vi "CRYAutoScale Change.vi"(9 "sOption":string, 10 "Graph VI Ref":refnum<vi>, 11 "sAction":string) -> ()   [LabVIEW 2013]
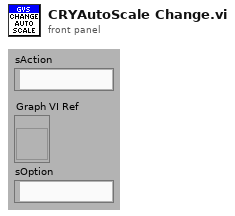
[diagram p1: front panel]
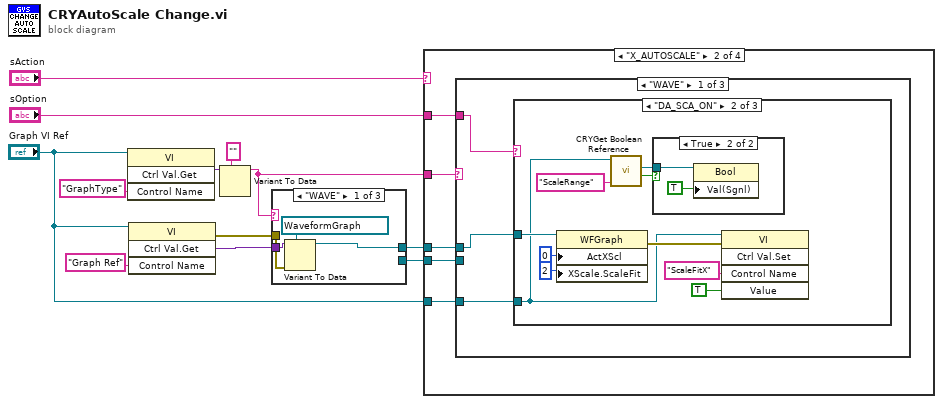
[diagram p0: block diagram]
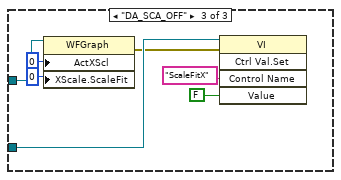
[diagram p5: hidden frame]
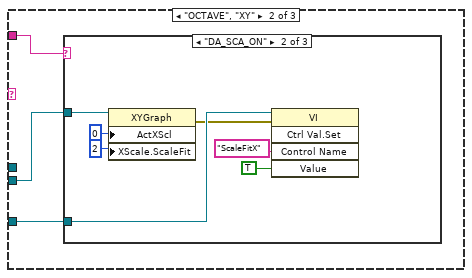
[diagram p6: hidden frame]
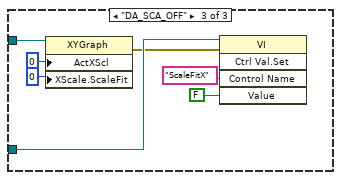
[diagram p8: hidden frame]
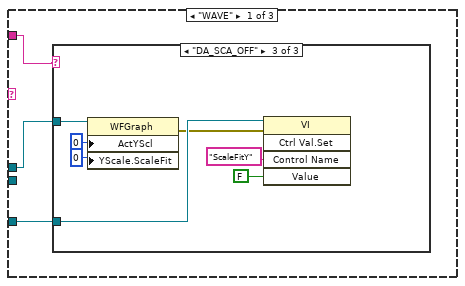
[diagram p11: hidden frame]
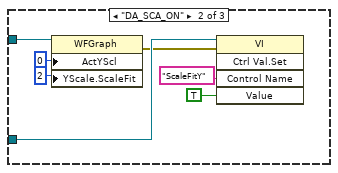
[diagram p13: hidden frame]
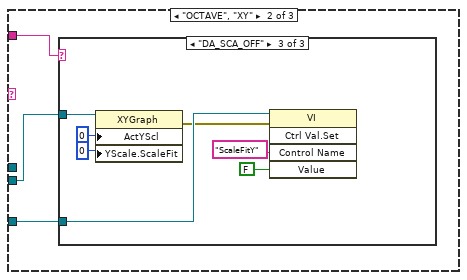
[diagram p14: hidden frame]
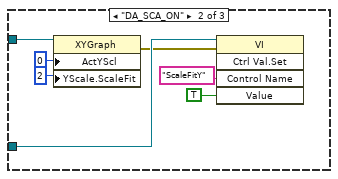
[diagram p16: hidden frame]
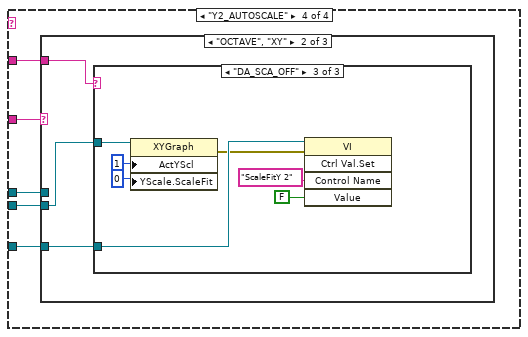
[diagram p17: hidden frame]
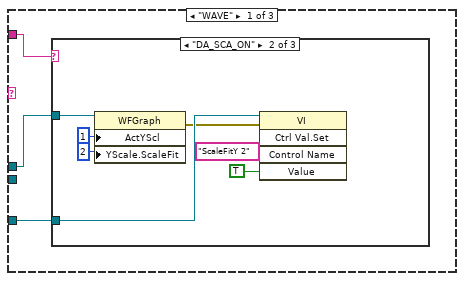
[diagram p18: hidden frame]
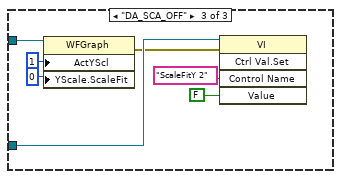
[diagram p20: hidden frame]
diagram:
  n1 = invoke class="VI" method="Ctrl Val.Get"(reference="Graph VI Ref", "Control Name"="GraphType") -> ("Get Control Value Variant"=w8:variant)  [unwired: 2 in, 3 out]
  n2 = invoke class="VI" method="Ctrl Val.Get"(reference="Graph VI Ref", "Control Name"="Graph Ref") -> (error out=w11:errorcluster, "Get Control Value Variant"=w12:variant)  [unwired: 2 in, 2 out]
  n3 = Variant To Data(type="" ("Control Name"), Variant=w8) -> (data=w4:string)  [unwired: 1 in, 1 out]
  n4 = case shown="\"WAVE\"" w4 {
    tunnel: w12 -> [w16 w20 _]
    tunnel: w11 -> [w15 w19 _]
    tunnel: [w13 _ _] -> w5
    tunnel: [_ w17 _] -> w3
    frame "WAVE" {
      n5 = Variant To Data(error in=w15, type=refnum<vi> refnum ("Legend Ref"), Variant=w16) -> (data=w13:refnum<vi>)  [unwired: 1 out]
    }
    frame "OCTAVE", "XY" {
      n6 = Variant To Data(error in=w19, type=refnum<vi> refnum ("Legend Ref"), Variant=w20) -> (data=w17:refnum<vi>)  [unwired: 1 out]
    }
    frame Default {
    }
  }
  n7 = case shown="\"X_AUTOSCALE\"" "sAction" {
    tunnel: w5 -> [_ w24 w68 w107]
    tunnel: w4 -> [_ w25 w69 w108]
    tunnel: w3 -> [_ w23 w67 w106]
    tunnel: "sOption" -> [_ w22 w66 w105]
    tunnel: "Graph VI Ref" -> [_ w21 w65 w104]
    frame Default {
    }
    frame "X_AUTOSCALE" {
      n8 = case shown="\"WAVE\"" w25 {
        tunnel: w24 -> [w27 _ _]
        tunnel: w23 -> [_ w50 _]
        tunnel: w22 -> [w28 w49 _]
        tunnel: w21 -> [w26 w48 _]
        frame "WAVE" {
          n9 = case shown="\"DA_SCA_ON\"" w28 {
            tunnel: w27 -> [_ w37 w45]
            tunnel: w26 -> [_ w32 w42]
            frame "NONE", Default {
            }
            frame "DA_SCA_ON" {
              n10 = property class="WFGraph"(reference=w37, "ActXScl"=0 ("Active X Scale"), "XScale.ScaleFit"=u8 2 ("t")) -> (error out=w33:errorcluster)  [unwired: 1 in, 1 out]
              n11 = call "CRYGet Boolean Reference.vi"("Label Name"="ScaleRange" ("Control Name"), "VI Refnum"=w32) -> ("Exist?"=w30:bool, "Boolean Ref"=w29:refnum<vi>)  [unwired: 7 in, 1 out]
              n12 = case shown="True" w30 {
                tunnel: w29 -> [_ w40]
                frame False {
                }
                frame True {
                  n13 = property class="Bool"(reference=w40, "Val(Sgnl)"=TRUE ("Visible")) -> ()  [unwired: 1 in, 2 out]
                }
              }
              n14 = invoke class="VI" method="Ctrl Val.Set"(reference=w32, error in=w33, "Control Name"="ScaleFitX", "Value"=TRUE ("Visible")) -> ()  [unwired: 1 in, 5 out]
            }
            frame "DA_SCA_OFF" {
              n15 = property class="WFGraph"(reference=w45, "ActXScl"=0 ("Active X Scale"), "XScale.ScaleFit"=u8 0 ("t")) -> (error out=w41:errorcluster)  [unwired: 1 in, 1 out]
              n16 = invoke class="VI" method="Ctrl Val.Set"(reference=w42, error in=w41, "Control Name"="ScaleFitX", "Value"=FALSE ("Visible")) -> ()  [unwired: 1 in, 5 out]
            }
          }
        }
        frame "OCTAVE", "XY" {
          n17 = case shown="\"DA_SCA_ON\"" w49 {
            tunnel: w50 -> [_ w56 w62]
            tunnel: w48 -> [_ w52 w59]
            frame "NONE", Default {
            }
            frame "DA_SCA_ON" {
              n18 = property class="XYGraph"(reference=w56, "ActXScl"=0 ("Active X Scale"), "XScale.ScaleFit"=u8 2 ("t")) -> (error out=w51:errorcluster)  [unwired: 1 in, 1 out]
              n19 = invoke class="VI" method="Ctrl Val.Set"(reference=w52, error in=w51, "Control Name"="ScaleFitX", "Value"=TRUE ("Visible")) -> ()  [unwired: 1 in, 5 out]
            }
            frame "DA_SCA_OFF" {
              n20 = property class="XYGraph"(reference=w62, "ActXScl"=0 ("Active X Scale"), "XScale.ScaleFit"=u8 0 ("t")) -> (error out=w58:errorcluster)  [unwired: 1 in, 1 out]
              n21 = invoke class="VI" method="Ctrl Val.Set"(reference=w59, error in=w58, "Control Name"="ScaleFitX", "Value"=FALSE ("Visible")) -> ()  [unwired: 1 in, 5 out]
            }
          }
        }
        frame Default {
        }
      }
    }
    frame "Y1_AUTOSCALE" {
      n22 = case shown="Default" w69 {
        tunnel: w68 -> [w71 _ _]
        tunnel: w67 -> [_ w87 _]
        tunnel: w66 -> [w72 w88 _]
        tunnel: w65 -> [w70 w89 _]
        frame "WAVE" {
          n23 = case shown="\"DA_SCA_OFF\"" w72 {
            tunnel: w71 -> [_ w78 w84]
            tunnel: w70 -> [_ w74 w81]
            frame "NONE", Default {
            }
            frame "DA_SCA_ON" {
              n24 = property class="WFGraph"(reference=w78, "ActYScl"=0 ("Active X Scale"), "YScale.ScaleFit"=u8 2 ("t")) -> (error out=w73:errorcluster)  [unwired: 1 in, 1 out]
              n25 = invoke class="VI" method="Ctrl Val.Set"(reference=w74, error in=w73, "Control Name"="ScaleFitY", "Value"=TRUE ("Visible")) -> ()  [unwired: 1 in, 5 out]
            }
            frame "DA_SCA_OFF" {
              n26 = property class="WFGraph"(reference=w84, "ActYScl"=0 ("Active X Scale"), "YScale.ScaleFit"=u8 0 ("t")) -> (error out=w80:errorcluster)  [unwired: 1 in, 1 out]
              n27 = invoke class="VI" method="Ctrl Val.Set"(reference=w81, error in=w80, "Control Name"="ScaleFitY", "Value"=FALSE ("Visible")) -> ()  [unwired: 1 in, 5 out]
            }
          }
        }
        frame "OCTAVE", "XY" {
          n28 = case shown="\"DA_SCA_OFF\"" w88 {
            tunnel: w87 -> [_ w95 w101]
            tunnel: w89 -> [_ w91 w98]
            frame "NONE", Default {
            }
            frame "DA_SCA_ON" {
              n29 = property class="XYGraph"(reference=w95, "ActYScl"=0 ("Active X Scale"), "YScale.ScaleFit"=u8 2 ("t")) -> (error out=w90:errorcluster)  [unwired: 1 in, 1 out]
              n30 = invoke class="VI" method="Ctrl Val.Set"(reference=w91, error in=w90, "Control Name"="ScaleFitY", "Value"=TRUE ("Visible")) -> ()  [unwired: 1 in, 5 out]
            }
            frame "DA_SCA_OFF" {
              n31 = property class="XYGraph"(reference=w101, "ActYScl"=0 ("Active X Scale"), "YScale.ScaleFit"=u8 0 ("t")) -> (error out=w97:errorcluster)  [unwired: 1 in, 1 out]
              n32 = invoke class="VI" method="Ctrl Val.Set"(reference=w98, error in=w97, "Control Name"="ScaleFitY", "Value"=FALSE ("Visible")) -> ()  [unwired: 1 in, 5 out]
            }
          }
        }
        frame Default {
        }
      }
    }
    frame "Y2_AUTOSCALE" {
      n33 = case shown="\"OCTAVE\", \"XY\"" w108 {
        tunnel: w107 -> [w110 _ _]
        tunnel: w106 -> [_ w127 _]
        tunnel: w105 -> [w111 w128 _]
        tunnel: w104 -> [w109 w126 _]
        frame "WAVE" {
          n34 = case shown="\"DA_SCA_ON\"" w111 {
            tunnel: w110 -> [_ w117 w123]
            tunnel: w109 -> [_ w113 w120]
            frame "NONE", Default {
            }
            frame "DA_SCA_ON" {
              n35 = property class="WFGraph"(reference=w117, "ActYScl"=1 ("Active X Scale"), "YScale.ScaleFit"=u8 2 ("t")) -> (error out=w112:errorcluster)  [unwired: 1 in, 1 out]
              n36 = invoke class="VI" method="Ctrl Val.Set"(reference=w113, error in=w112, "Control Name"="ScaleFitY 2", "Value"=TRUE ("Visible")) -> ()  [unwired: 1 in, 5 out]
            }
            frame "DA_SCA_OFF" {
              n37 = property class="WFGraph"(reference=w123, "ActYScl"=1 ("Active X Scale"), "YScale.ScaleFit"=u8 0 ("t")) -> (error out=w119:errorcluster)  [unwired: 1 in, 1 out]
              n38 = invoke class="VI" method="Ctrl Val.Set"(reference=w120, error in=w119, "Control Name"="ScaleFitY 2", "Value"=FALSE ("Visible")) -> ()  [unwired: 1 in, 5 out]
            }
          }
        }
        frame "OCTAVE", "XY" {
          n39 = case shown="\"DA_SCA_OFF\"" w128 {
            tunnel: w127 -> [_ w134 w140]
            tunnel: w126 -> [_ w130 w137]
            frame "NONE", Default {
            }
            frame "DA_SCA_ON" {
              n40 = property class="XYGraph"(reference=w134, "ActYScl"=1 ("Active X Scale"), "YScale.ScaleFit"=u8 2 ("t")) -> (error out=w129:errorcluster)  [unwired: 1 in, 1 out]
              n41 = invoke class="VI" method="Ctrl Val.Set"(reference=w130, error in=w129, "Control Name"="ScaleFitY 2", "Value"=TRUE ("Visible")) -> ()  [unwired: 1 in, 5 out]
            }
            frame "DA_SCA_OFF" {
              n42 = property class="XYGraph"(reference=w140, "ActYScl"=1 ("Active X Scale"), "YScale.ScaleFit"=u8 0 ("t")) -> (error out=w136:errorcluster)  [unwired: 1 in, 1 out]
              n43 = invoke class="VI" method="Ctrl Val.Set"(reference=w137, error in=w136, "Control Name"="ScaleFitY 2", "Value"=FALSE ("Visible")) -> ()  [unwired: 1 in, 5 out]
            }
          }
        }
        frame Default {
        }
      }
    }
  }
